vi "MH_GetHardwareInfo.vi"(8 "error in (no error)":errorcluster, 11 "devidx":i32) -> (0 "error out":errorcluster, 1 "Partnum":string, 2 "Model":string, 3 "return type":i32, 4 "Version":string)   [LabVIEW 2019]
uses:
  <userlib>/MultiHarp150/MH_DllPath_global.vi
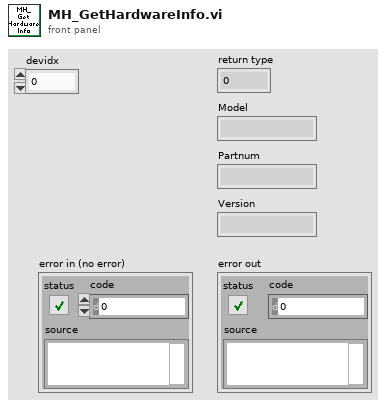
[diagram p1: front panel]
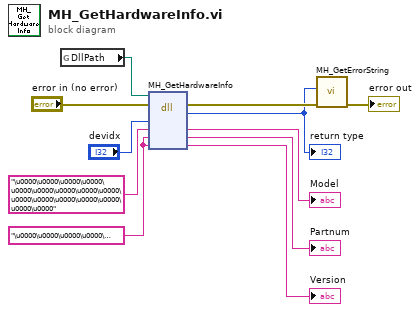
[diagram p0: block diagram]
diagram:
  w5 = "\u0000\u0000\u0000\u0000\u0000\u0000\u0000\u0000" ("Model")
  n1 = global read "MH_DllPath_global.vi" "DllPath"() -> (w10:path)
  n2 = dll-call lib="MHLib64.dll" fn="MH_GetHardwareInfo"(path in=w10, error in="error in (no error)", "devidx"="devidx", "Model"="\u0000\u0000\u0000\u0000\u0000\u0000\u0000\u0000\u0000\u0000\u0000\u0000\u0000\u0000\u0000\u0000", "Partnum"=w5, "Version"=w5) -> (error out=w8:errorcluster, "return type"=w7:i32, "Model"=→"Model":string, "Partnum"=→"Partnum":string, "Version"=→"Version":string)  [unwired: 2 in, 1 out]
  "return type" <- w7
  n3 = call <userlib>:"MH_GetErrorString.vi"("error in (no error)"=w8, "code"=w7) -> ("error out"=→"error out":errorcluster)  [unwired: 7 in, 2 out]
